vi "Master Setup Titles.vi"() -> (0 "Sorted Titles Indices":i32[](array[numeric]), 1 "Setup Patterns":string[](array[string]), 2 "Setup Description":string[](array[string]), 3 "Setup Description w/Numbers":string[](array[string]), 4 "Sorted Setup Description":string[](array[string]), 6 "Sorted Setup Patterns":string[](array[string]))   [LabVIEW 2017]
uses:
  My Global Var.vi
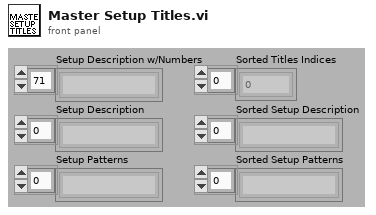
[diagram p1: front panel]
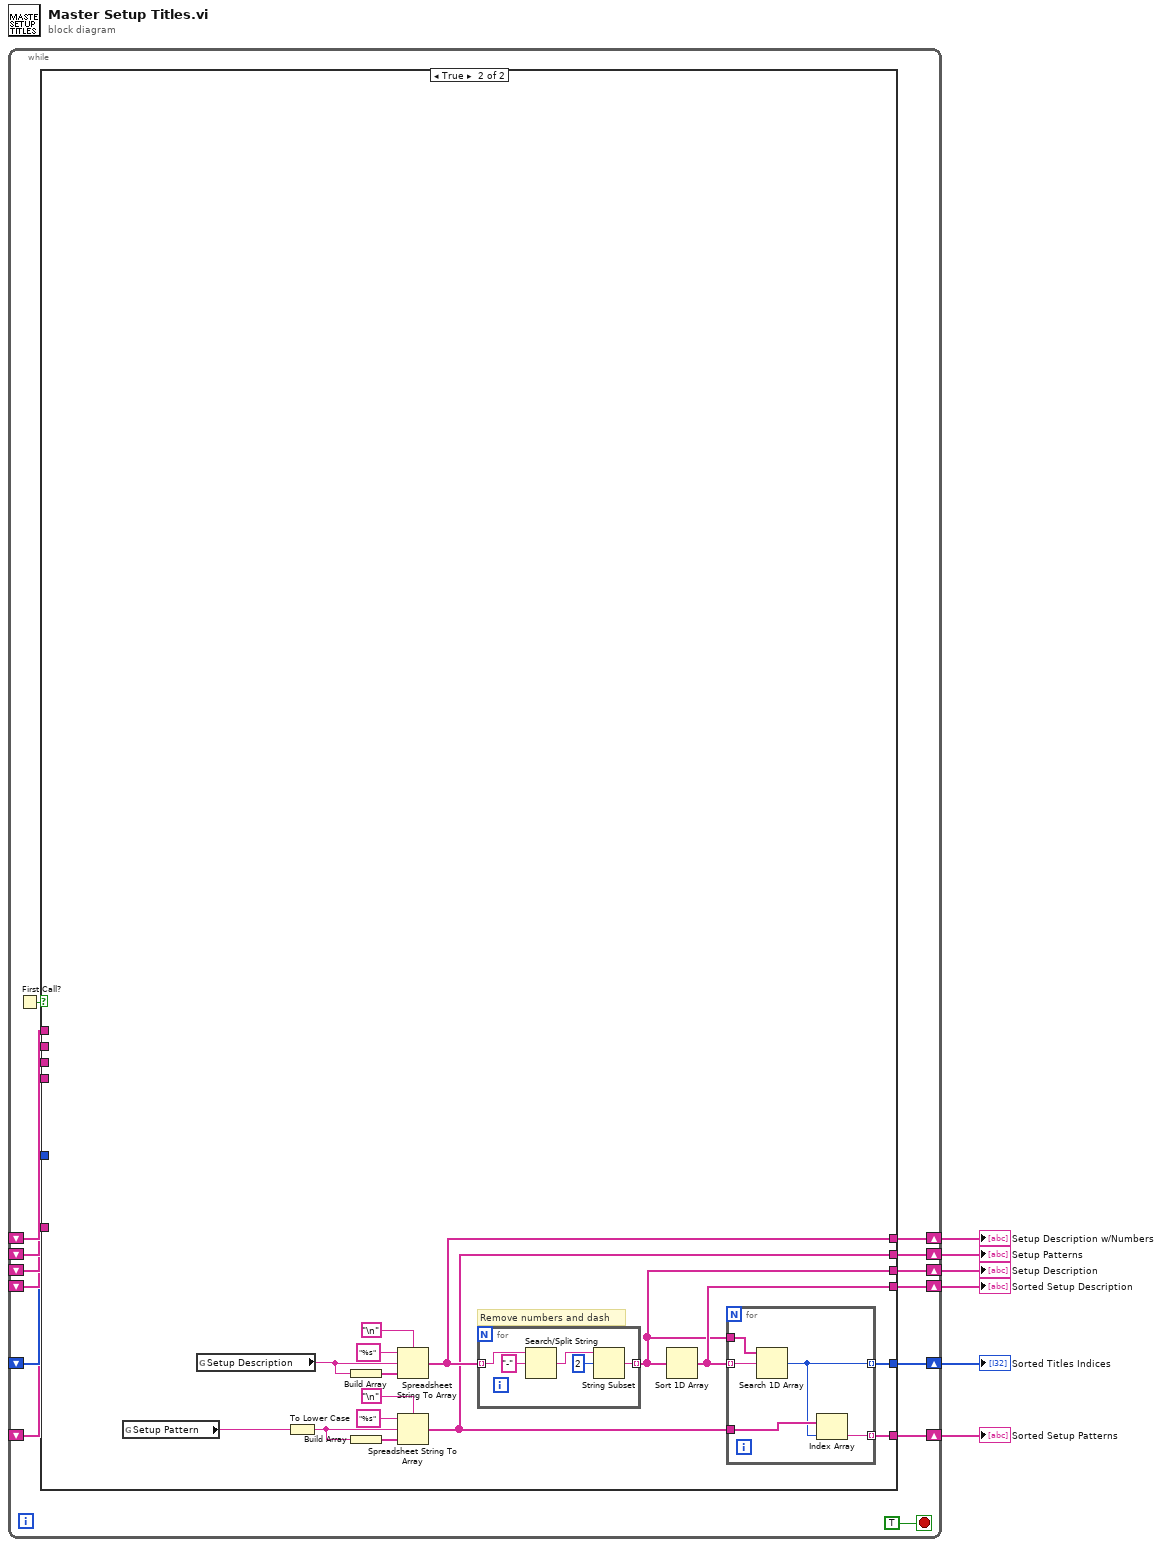
[diagram p0: block diagram]
diagram:
  n1 = while {
    shift-right: [w20] -> w6
    shift-left: _ -> [w13]
    shift-right: [w17] -> w3
    shift-left: _ -> [w12]
    shift-right: [w18] -> w4
    shift-left: _ -> [w11]
    shift-right: [w19] -> w5
    shift-left: _ -> [w10]
    shift-right: [w16] -> w2
    shift-left: _ -> [w9]
    shift-right: [w15] -> w1
    shift-left: _ -> [w8]
    stop <- TRUE stop-if-true
    n2 = First Call?() -> (First Call?: T/F=w14:bool)
    n3 = case shown="True" w14 {
      tunnel: [w26 w40] -> w20
      tunnel: [w23 w34] -> w19
      tunnel: [w24 w33] -> w18
      tunnel: [w25 w32] -> w17
      tunnel: [w22 w31] -> w16
      tunnel: [w21 w30] -> w15
      tunnel: w13 -> [w26 _]
      tunnel: w12 -> [w25 _]
      tunnel: w11 -> [w24 _]
      tunnel: w10 -> [w23 _]
      tunnel: w9 -> [w22 _]
      tunnel: w8 -> [w21 _]
      frame False {
      }
      frame True {
        # "Remove numbers and dash"
        n4 = global read "My Global Var.vi" "Setup Pattern"() -> (w28:string)
        n5 = global read "My Global Var.vi" "Setup Description"() -> (w27:string)
        n6 = To Lower Case(string=w28) -> (all lower case string=w41:string)
        n7 = Build Array(w27) -> (w35:string[])
        n8 = Build Array(w41) -> (w39:string[])
        n9 = Spreadsheet String To Array(delimiter (Tab)="\n", format string="%s", spreadsheet string=w27, array type (2D Dbl)=w35) -> (array=w40:string[])
        n10 = Spreadsheet String To Array(delimiter (Tab)="\n", format string="%s", spreadsheet string=w41, array type (2D Dbl)=w39) -> (array=w32:string[])
        n11 = for {
          tunnel: w40 -> [w51] mode=indexing
          tunnel: [w47] -> w33 mode=indexing
          n12 = Search/Split String(string=w51, search string/char (-)="-") -> (match + rest of string=w49:string)  [unwired: 1 in, 2 out]
          n13 = String Subset(string=w49, offset (0)=2) -> (substring=w47:string)  [unwired: 1 in]
        }
        n14 = Sort 1D Array(array=w33) -> (sorted array=w34:string[])
        n15 = for {
          tunnel: w34 -> [w45] mode=indexing
          tunnel: w33 -> [w46]
          tunnel: [w43] -> w31 mode=indexing
          tunnel: w32 -> [w44]
          tunnel: [w42] -> w30 mode=indexing
          n16 = Search 1D Array(1D array=w46, element=w45) -> (index of element=w43:i32)  [unwired: 1 in]
          n17 = Index Array(array=w44, index=w43) -> (element=w42:string)
        }
      }
    }
  }
  "Setup Description" <- w4
  "Setup Description w/Numbers" <- w6
  "Setup Patterns" <- w3
  "Sorted Setup Description" <- w5
  "Sorted Titles Indices" <- w2
  "Sorted Setup Patterns" <- w1
